vi "Read Tree Item Open State.vi"(8 "error in (no error)":errorcluster, 11 "File Explorer in":refnum<class "File Explorer.lvclass">) -> (0 "error out":errorcluster, 3 "File Explorer out":refnum<class "File Explorer.lvclass">)   [LabVIEW 2020, in "File Explorer.lvlib" / "File Explorer.lvclass"]
uses:
  <vilib>/gpm_packages/@cs/file-explorer-extension/Source/File Explorer/File Explorer/File Explorer.lvclass
  <vilib>/gpm_packages/@cs/file-explorer-extension/Source/File Explorer/File Explorer/File Explorer.lvclass/File Explorer.ctl
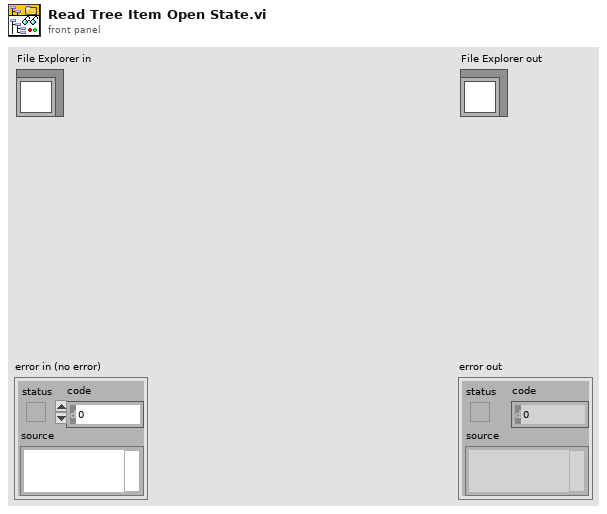
[diagram p1: front panel]
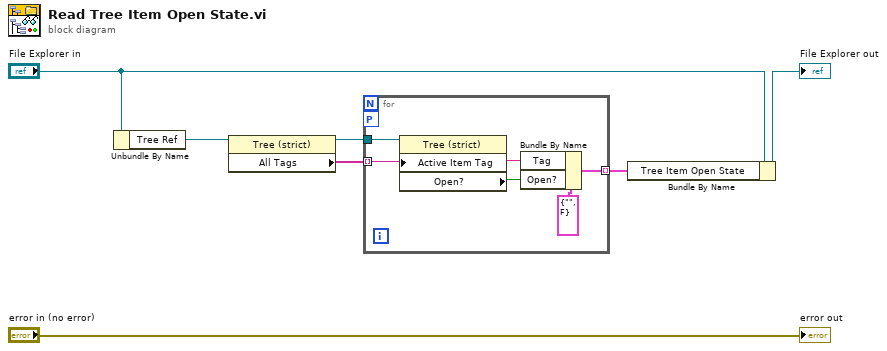
[diagram p0: block diagram]
diagram:
  n1 = Unbundle By Name("File Explorer in") -> ("Tree Ref"=w6:refnum<vi>)
  n2 = property class="Tree (strict)"(reference=w6) -> (reference out=w5:refnum<vi>, "All Tags"=w4:string[])  [unwired: 1 in, 1 out]
  n3 = for {
    tunnel: w4 -> [w10] mode=indexing
    tunnel: [w8] -> w1 mode=indexing
    tunnel: w5 -> [w12]
    workers-P: _ -> [_]
    n4 = property class="Tree (strict)"(reference=w12, "Active Item Tag"=w10) -> ("Open?"=w9:bool)  [unwired: 1 in, 2 out]
    n5 = Bundle By Name(cluster=cluster{"Tag":string, "Open?":bool} {"Tag"="", "Open?"=FALSE} ("Item Open State"), "Tag"=w10, "Open?"=w9) -> (w8:cluster{"Tag":string, "Open?":bool})
  }
  n6 = Bundle By Name(cluster="File Explorer in", "Tree Item Open State"=w1) -> (→"File Explorer out":refnum<class "File Explorer.lvclass">)
  "error out" <- "error in (no error)"
